vi "ShapeDetectResultTable.vi"(7 "Table":refnum<vi>, 8 "error in (no error)":errorcluster, 10 "Result":variant, 11 "Shape Type":T2(ring)) -> (0 "error out":errorcluster)   [LabVIEW 2019]
uses:
  Controls/ShapeDectect/V_ShapeDectectFinalResult.ctl
panel:
  in  "Shapedectect Result Out":T1
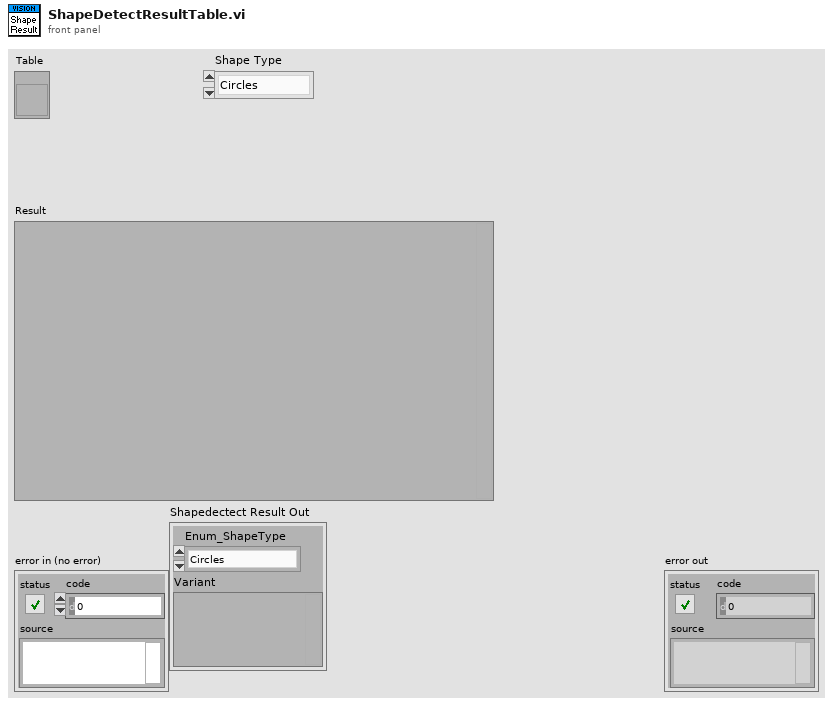
[diagram p1: front panel]
types:
  T1 = typedef "V_ShapeDectectFinalResult.ctl" = cluster{"Enum_ShapeType":enum16{"Circles", "Ellipses", "Lines", "Rectangles"}, "Variant":variant}
  T2 = enum16{"Circles", "Ellipses", "Lines", "Rectangles"}
  T3 = cluster{"Circles":cluster{"Position":cluster{"X":sgl, "Y":sgl}, "Radius":dbl, "Score":dbl}[], "Circles (Calibrated)":cluster{"Position":cluster{"X":sgl, "Y":sgl}, "Radius":dbl, "Score":dbl}[]}
  T4 = cluster{"Position":cluster{"X":sgl, "Y":sgl}, "Radius":dbl, "Score":dbl}[]
  T5 = cluster{"Pixel":cluster{"Position":cluster{"X":sgl, "Y":sgl}, "Angle":dbl, "Major Radius":dbl, "Minor Radius":dbl, "Score":dbl}[], "Ellipses (Calibrated)":cluster{"Position":cluster{"X":sgl, "Y":sgl}, "Orientation":dbl, "Major Radius":dbl, "Minor Radius":dbl, "Score":dbl}[]}
  T6 = cluster{"Position":cluster{"X":sgl, "Y":sgl}, "Angle":dbl, "Major Radius":dbl, "Minor Radius":dbl, "Score":dbl}[]
  T7 = cluster{"Lines":cluster{"Start Point":cluster{"X":sgl, "Y":sgl}, "End Point":cluster{"X":sgl, "Y":sgl}, "Length":dbl, "Angle":dbl, "Score":dbl}[], "Lines Calibrated":cluster{"Start Point":cluster{"X":sgl, "Y":sgl}, "End Point":cluster{"X":sgl, "Y":sgl}, "Length":dbl, "Orientation":dbl, "Score":dbl}[]}
  T8 = cluster{"Start Point":cluster{"X":sgl, "Y":sgl}, "End Point":cluster{"X":sgl, "Y":sgl}, "Length":dbl, "Angle":dbl, "Score":dbl}[]
  T9 = cluster{"Rectangles":cluster{"Corners":cluster{"X":sgl, "Y":sgl}[], "Angle":dbl, "Width":dbl, "Height":dbl, "Score":dbl}[], "Rectangles Calibrated":cluster{"Corners":cluster{"X":sgl, "Y":sgl}[], "Angle":dbl, "Width":dbl, "Height":dbl, "Score":dbl}[]}
  T10 = cluster{"Corners":cluster{"X":sgl, "Y":sgl}[], "Angle":dbl, "Width":dbl, "Height":dbl, "Score":dbl}[]
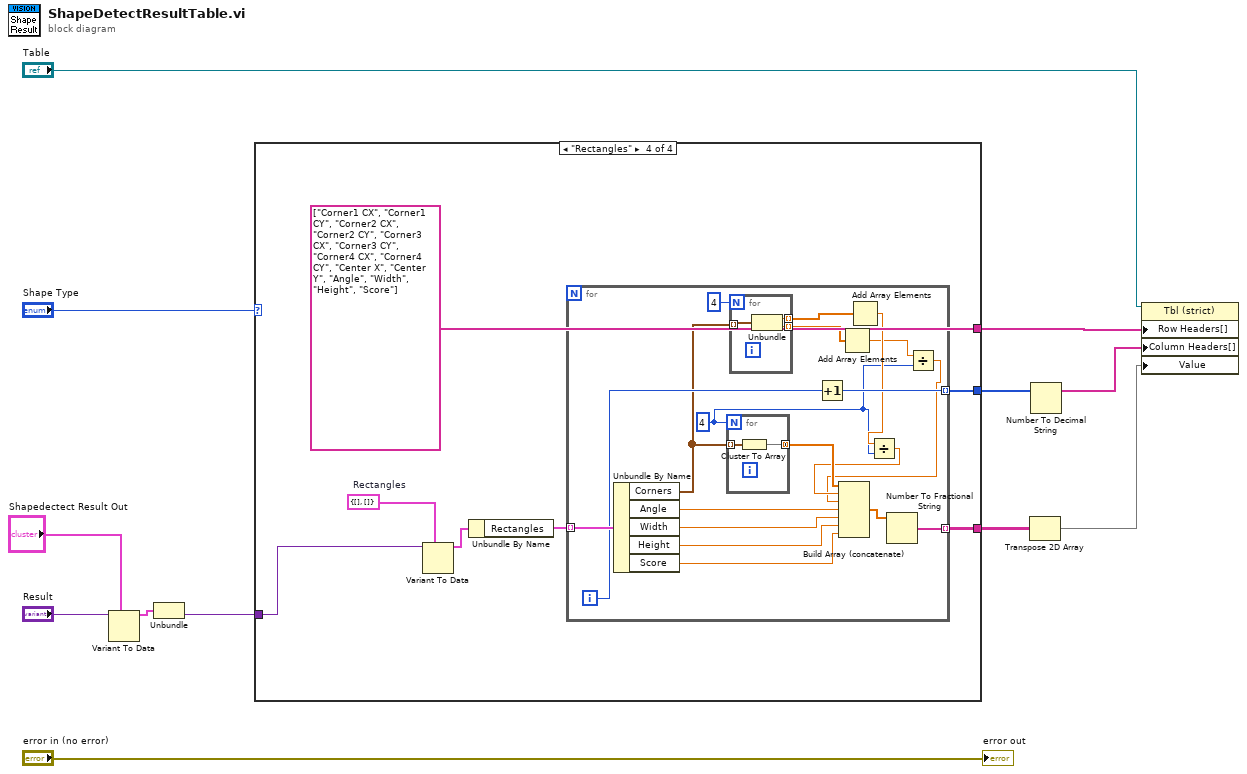
[diagram p0: block diagram]
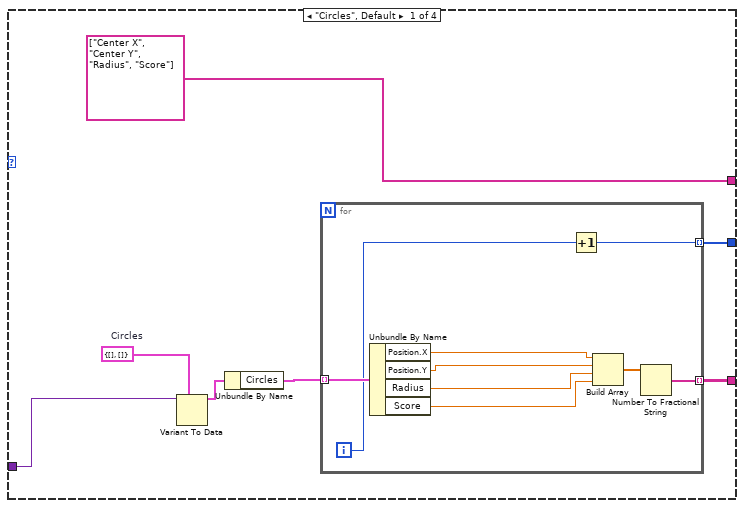
[diagram p2: hidden frame]
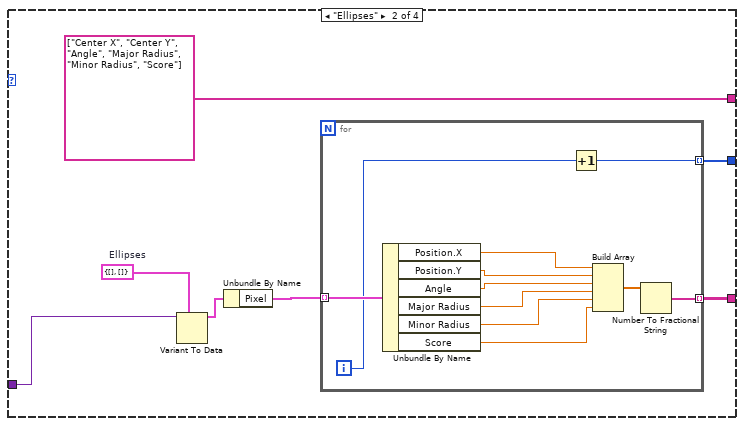
[diagram p3: hidden frame]
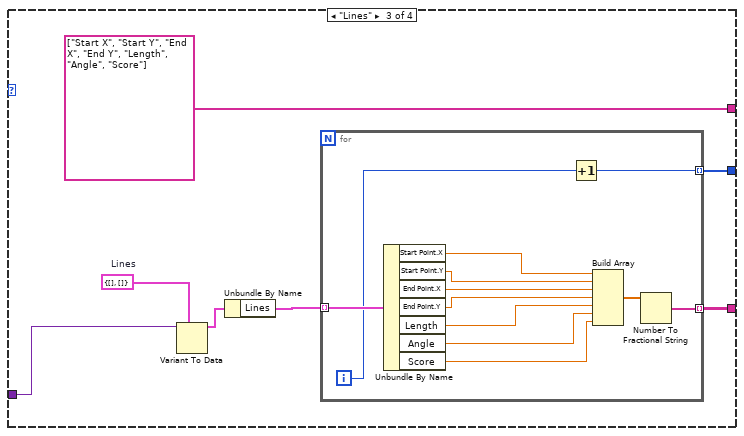
[diagram p4: hidden frame]
diagram:
  n1 = Variant To Data(type="Shapedectect Result Out", Variant="Result") -> (data=w2:T1)  [unwired: 1 in, 1 out]
  n2 = Unbundle(w2) -> ("Variant"=w1:variant)  [unwired: 1 out]
  n3 = case shown="\"Rectangles\"" "Shape Type" {
    tunnel: [string[] ["Center X", "Center Y", "Radius", "Score"] string[] ["Center X", "Center Y", "Angle", "Major Radius", "Minor Radius", "Score"] string[] ["Start X", "Start Y", "End X", "End Y", "Length", "Angle", "Score"] string[] ["Corner1 CX", "Corner1 CY", "Corner2 CX", "Corner2 CY", "Corner3 CX", "Corner3 CY", "Corner4 CX", "Corner4 CY", "Center X", "Center Y", "Angle", "Width", "Height", "Score"]] -> w10
    tunnel: w1 -> [w18 w33 w52 w69]
    tunnel: [w14 w30 w47 w67] -> w9
    tunnel: [w13 w29 w48 w66] -> w5
    frame "Circles", Default {
      w17 = T3 {"Circles"=[], "Circles (Calibrated)"=[]}  # Circles
      n4 = Variant To Data(type=w17, Variant=w18) -> (data=w16:T3)  [unwired: 1 in, 1 out]
      n5 = Unbundle By Name(w16) -> ("Circles"=w15:T4)
      n6 = for {
        tunnel: w15 -> [w28] mode=indexing
        tunnel: [w23] -> w14 mode=indexing
        tunnel: [w21] -> w13 mode=indexing
        i -> [w22]
        n7 = Unbundle By Name(w28) -> ("Position.X"=w20:sgl, "Position.Y"=w27:sgl, "Radius"=w25:dbl, "Score"=w26:dbl)
        n8 = Increment(x=w22) -> (x+1=w21:i32)
        n9 = Build Array(w20, w27, w25, w26) -> (w24:dbl[])
        n10 = Number To Fractional String(number=w24) -> (F-format string=w23:string[])  [unwired: 3 in]
      }
    }
    frame "Ellipses" {
      w34 = T5 {"Pixel"=[], "Ellipses (Calibrated)"=[]}  # Ellipses
      n11 = Variant To Data(type=w34, Variant=w33) -> (data=w32:T5)  [unwired: 1 in, 1 out]
      n12 = Unbundle By Name(w32) -> ("Pixel"=w31:T6)
      n13 = for {
        tunnel: w31 -> [w46] mode=indexing
        tunnel: [w42] -> w30 mode=indexing
        tunnel: [w40] -> w29 mode=indexing
        i -> [w41]
        n14 = Unbundle By Name(w46) -> ("Position.X"=w39:sgl, "Position.Y"=w45:sgl, "Angle"=w44:dbl, "Major Radius"=w37:dbl, "Minor Radius"=w36:dbl, "Score"=w38:dbl)
        n15 = Increment(x=w41) -> (x+1=w40:i32)
        n16 = Build Array(w39, w45, w44, w37, w36, w38) -> (w43:dbl[])
        n17 = Number To Fractional String(number=w43) -> (F-format string=w42:string[])  [unwired: 3 in]
      }
    }
    frame "Lines" {
      w51 = T7 {"Lines"=[], "Lines Calibrated"=[]}  # Lines
      n18 = Variant To Data(type=w51, Variant=w52) -> (data=w50:T7)  [unwired: 1 in, 1 out]
      n19 = Unbundle By Name(w50) -> ("Lines"=w49:T8)
      n20 = for {
        tunnel: w49 -> [w65] mode=indexing
        tunnel: [w61] -> w47 mode=indexing
        tunnel: [w59] -> w48 mode=indexing
        i -> [w60]
        n21 = Unbundle By Name(w65) -> ("Start Point.X"=w55:sgl, "Start Point.Y"=w64:sgl, "End Point.X"=w63:sgl, "End Point.Y"=w57:sgl, "Length"=w56:dbl, "Angle"=w58:dbl, "Score"=w54:dbl)
        n22 = Increment(x=w60) -> (x+1=w59:i32)
        n23 = Build Array(w55, w64, w63, w57, w56, w58, w54) -> (w62:dbl[])
        n24 = Number To Fractional String(number=w62) -> (F-format string=w61:string[])  [unwired: 3 in]
      }
    }
    frame "Rectangles" {
      w70 = T9 {"Rectangles"=[], "Rectangles Calibrated"=[]}  # Rectangles
      n25 = Variant To Data(type=w70, Variant=w69) -> (data=w68:T9)  [unwired: 1 in, 1 out]
      n26 = Unbundle By Name(w68) -> ("Rectangles"=w71:T10)
      n27 = for {
        tunnel: w71 -> [w91] mode=indexing
        tunnel: [w85] -> w67 mode=indexing
        tunnel: [w83] -> w66 mode=indexing
        i -> [w84]
        w73 = 4
        n28 = Unbundle By Name(w91) -> ("Corners"=w82:cluster{"X":sgl, "Y":sgl}[], "Angle"=w90:dbl, "Width"=w87:dbl, "Height"=w88:dbl, "Score"=w89:dbl)
        n29 = for {
          N: w73 -> [_]
          tunnel: w82 -> [w96] mode=indexing
          tunnel: [w95] -> w76 mode=concatenating
          n30 = Cluster To Array(cluster=w96) -> (array=w95:sgl[])
        }
        n31 = for {
          N: 4 -> [_]
          tunnel: w82 -> [w94] mode=indexing
          tunnel: [w93] -> w80 mode=indexing
          tunnel: [w92] -> w79 mode=indexing
          n32 = Unbundle(w94) -> ("X"=w93:sgl, "Y"=w92:sgl)
        }
        n33 = Increment(x=w84) -> (x+1=w83:i32)
        n34 = Add Array Elements(numeric array=w79) -> (sum=w77:sgl)
        n35 = Add Array Elements(numeric array=w80) -> (sum=w78:sgl)
        n36 = Divide(x=w78, y=w73) -> (x/y=w75:sgl)
        n37 = Divide(x=w77, y=w73) -> (x/y=w74:sgl)
        n38 = Build Array (concatenate)(w76, w75, w74, w90, w87, w88, w89) -> (w86:dbl[])
        n39 = Number To Fractional String(number=w86) -> (F-format string=w85:string[])  [unwired: 3 in]
      }
    }
  }
  n40 = Transpose 2D Array(2D array=w9) -> (transposed array=w7:string[][])
  n41 = Number To Decimal String(number=w5) -> (decimal integer string=w6:string[])  [unwired: 1 in]
  n42 = property class="Tbl (strict)"(reference="Table", "Row Headers[]"=w10, "Column Headers[]"=w6, "Value"=w7) -> ()  [unwired: 1 in, 2 out]
  "error out" <- "error in (no error)"
